vi "Decimate and Filter.vi"(6 "Enabled?":bool, 8 "error in (no error)":errorcluster, 9 "low cutoff freq: fl":dbl, 10 "decimating factor":i32, 11 "Waveform in":waveform(dbl)) -> (0 "error out":errorcluster, 3 "Decimated and Filtered Array":dbl[](array[numeric]))   [LabVIEW 2016, in "Transport.lvclass"]
uses:
  Transport.lvclass
  <vilib>/Analysis/NI_AALBase.lvlib
  <vilib>/Analysis/3filter.llb/Butterworth Filter (DBL).vi
  <vilib>/Analysis/3filter.llb/Filter Passband Type.ctl
  <vilib>/Analysis/NI_AALPro.lvlib
  <vilib>/Analysis/2dsp.llb/Decimate (single shot, DBL).vi
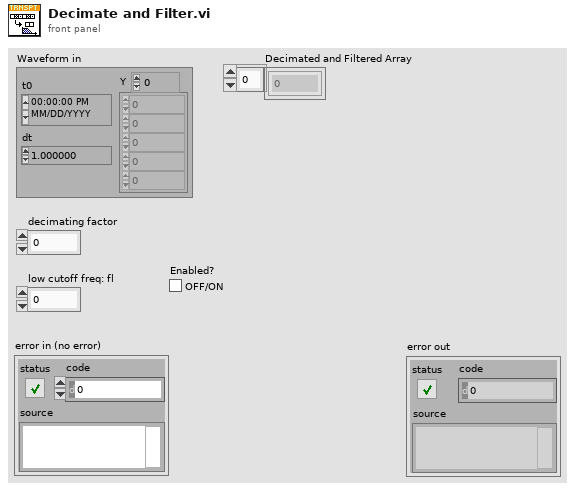
[diagram p1: front panel]
types:
  T1 = typedef "NI_AALBase.lvlib/Filter Passband Type.ctl" = enum32{"Lowpass", "Highpass", "Bandpass", "Bandstop"}
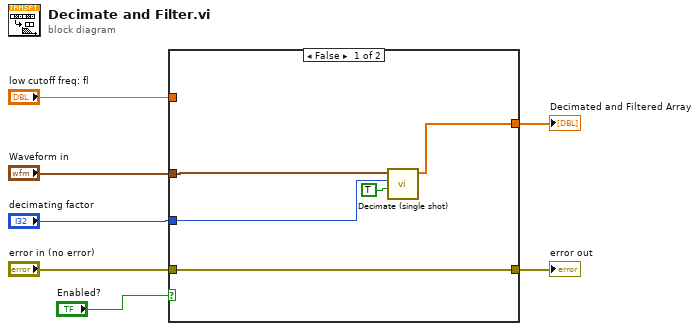
[diagram p0: block diagram]
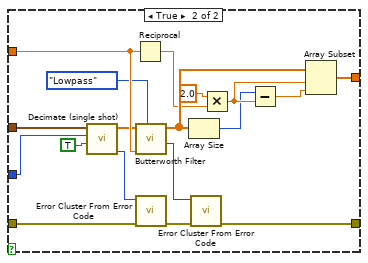
[diagram p2: hidden frame]
diagram:
  n1 = case shown="False" "Enabled?" {
    tunnel: "low cutoff freq: fl" -> [_ w30]
    tunnel: [w8 w29] -> w6
    tunnel: "Waveform in" -> [w10 w27]
    tunnel: [w12 w15] -> w4
    tunnel: "error in (no error)" -> [w12 w14]
    tunnel: "decimating factor" -> [w9 w13]
    frame False {
      n2 = call-poly <vilib>:"Decimate (single shot).vi"("averaging"=TRUE, "decimating factor"=w9, "X"=w10) -> ("Decimated Array"=w8:dbl[])  [unwired: 7 in, 1 out]
    }
    frame True {
      n3 = call-poly <vilib>:"Decimate (single shot).vi"("averaging"=TRUE, "decimating factor"=w13, "X"=w27) -> ("error"=w18:i32, "Decimated Array"=w26:dbl[])  [unwired: 7 in]
      n4 = Reciprocal(x=w30) -> (1/x=w21:dbl)
      n5 = call-poly <vilib>:"Butterworth Filter.vi"("filter type"=Filter_Passband_Type."Lowpass", "low cutoff freq: fl"=w30, "X"=w26) -> ("error"=w17:i32, "Filtered X"=w23:dbl[])  [unwired: 5 in]
      n6 = call <vilib>:"Error Cluster From Error Code.vi"("error in (no error)"=w14, "error code (0)"=w18) -> ("error out"=w16:errorcluster)  [unwired: 7 in]
      n7 = Array Size(array=w23) -> (size(s)=w20:i32)
      n8 = call <vilib>:"Error Cluster From Error Code.vi"("error in (no error)"=w16, "error code (0)"=w17) -> ("error out"=w15:errorcluster)  [unwired: 7 in]
      n9 = Multiply(x=2.0, y=w21) -> (x*y=w24:dbl)
      n10 = Subtract(x=w20, y=w24) -> (x-y=w28:dbl)
      n11 = Array Subset(array=w23, index=w24, length=w28) -> (w29:dbl[])
    }
  }
  "Decimated and Filtered Array" <- w6
  "error out" <- w4
